vi "Partial Fraction Expansion.vi"(8 "option":u16(ring) items=["Cancel Co-factors", "Reserve Co-factors"], 9 "tolerance":dbl=1e-05, 10 "Denominator":cdb[](array[numeric]) format="%#.6g", 11 "Numerator":cdb[](array[numeric]) format="%#.6g") -> (0 "error":i32, 1 "Residues":cdb[][](array[numeric]) format="%#.6g", 2 "Poles":cdb[](array[numeric]) format="%#.6g", 3 "Polynomial":cdb[](array[numeric]) format="%#.6g", 5 "Multiplicity":i32[](array[numeric]))   [LabVIEW 2010, in "NI_AALPro.lvlib"]
doc: "Calculates the partial fraction expansion of a polynomial using the Heaviside cover-up method."
uses:
  NI_AALPro.lvlib
  Remove Zero Coefficients (CDB).vi
  Divide Polynomials (CDB).vi
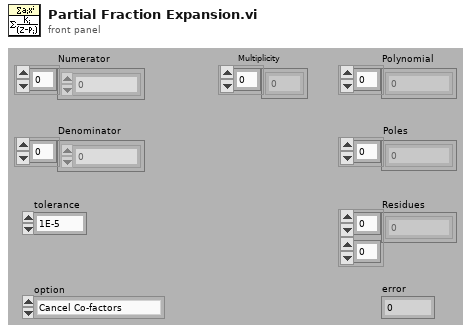
[diagram p1: front panel]
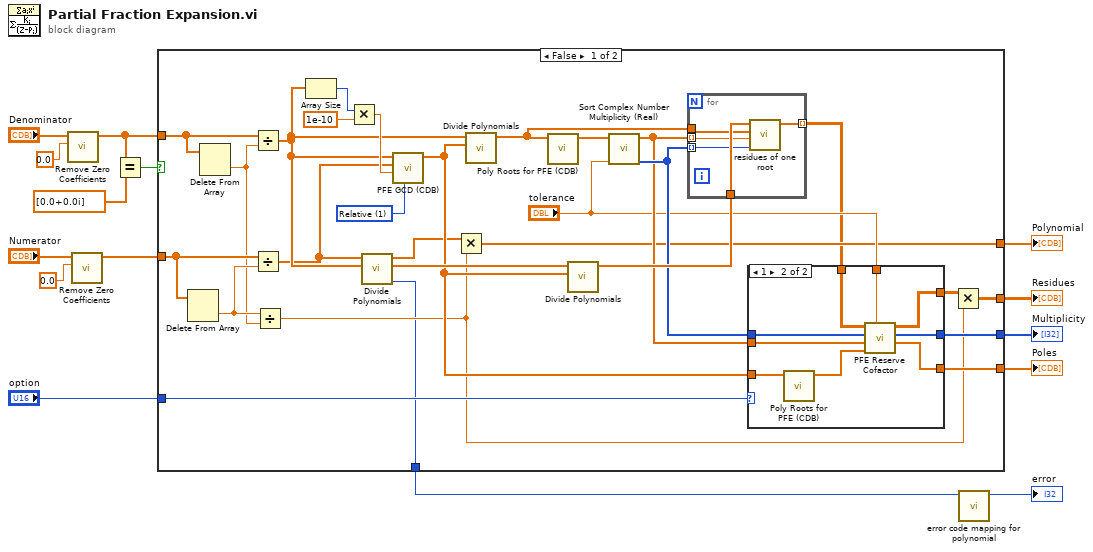
[diagram p0: block diagram]
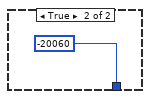
[diagram p3: hidden frame]
diagram:
  n1 = call-poly "Remove Zero Coefficients.vi"("threshold"=0.0, "P(x) In"="Denominator") -> ("P(x) Out"=w2:cdb[])  [unwired: 7 in, 2 out]
  n2 = call-poly "Remove Zero Coefficients.vi"("threshold"=0.0, "P(x) In"="Numerator") -> ("P(x) Out"=w8:cdb[])  [unwired: 7 in, 2 out]
  n3 = Equal?(x=w2, y=cdb[] [0.0+0.0i] ("P(x) Out")) -> (x = y?=w3:bool)
  n4 = case shown="False" w3 {
    tunnel: "option" -> [w39 _]
    tunnel: [w36 _] -> w10
    tunnel: [w35 _] -> w9
    tunnel: w2 -> [w29 _]
    tunnel: w8 -> [w27 _]
    tunnel: [w23 _] -> w7
    tunnel: [w17 _] -> w6
    tunnel: [w16 -20060] -> w4
    frame False {
      w30 = u16 1 items=["Absolute", "Relative"] ("tolerance type")
      n5 = Delete From Array(array=w27) -> (deleted portion=w25:cdb)  [unwired: 2 in, 1 out]
      n6 = Delete From Array(array=w29) -> (deleted portion=w24:cdb)  [unwired: 2 in, 1 out]
      n7 = Divide(x=w29, y=w24) -> (x/y=w28:cdb[])
      n8 = Divide(x=w27, y=w25) -> (x/y=w26:cdb[])
      n9 = Divide(x=w25, y=w24) -> (x/y=w18:cdb)
      n10 = Array Size(array=w28) -> (size(s)=w42:i32)
      n11 = Multiply(x=w42, y=1e-10 ("eps for GCD")) -> (x*y=w32:dbl)
      n12 = call-poly "Divide Polynomials.vi"("Q(x)"=w28, "P(x)"=w26) -> ("error"=w16:i32, "Remainder"=w41:cdb[], "P(x)/Q(x)"=w22:cdb[])  [unwired: 7 in]
      n13 = call "PFE GCD (CDB).vi"("tolerance type"=w30, "tolerance"=w32, "Q(x)"=w26, "P(x)"=w28) -> ("Greatest Common Divisor"=w31:cdb[])  [unwired: 6 in, 1 out]
      n14 = Multiply(x=w22, y=w18) -> (x*y=w23:cdb[])
      n15 = call-poly "Divide Polynomials.vi"("Q(x)"=w31, "P(x)"=w28) -> ("P(x)/Q(x)"=w21:cdb[])  [unwired: 7 in, 2 out]
      n16 = call "Poly Roots for PFE (CDB).vi"("P(x)"=w21) -> ("Roots"=w33:cdb[])  [unwired: 10 in]
      n17 = call-poly "Divide Polynomials.vi"("Q(x)"=w31, "P(x)"=w41) -> ("P(x)/Q(x)"=w40:cdb[])  [unwired: 7 in, 2 out]
      n18 = call "Sort Complex Number Multiplicity (Real).vi"("tolerance"="tolerance", "Complex numbers"=w33) -> ("Multiplicity"=w38:i32[], "Sorted unique complex numbers"=w37:cdb[])  [unwired: 8 in]
      n19 = for {
        tunnel: w38 -> [w57] mode=indexing
        tunnel: w37 -> [w58] mode=indexing
        tunnel: w40 -> [w60]
        tunnel: w21 -> [w59]
        tunnel: [w56] -> w20 mode=indexing
        n20 = call "residues of one root.vi"("multiplicity of root"=w57, "root"=w58, "Denominator"=w59, "Rest"=w60) -> ("Residues of root"=w56:cdb[])  [unwired: 7 in]
      }
      n21 = case shown="1" w39 {
        tunnel: w38 -> [w46 w54]
        tunnel: w37 -> [w45 w55]
        tunnel: [w45 w49] -> w36
        tunnel: [w46 w50] -> w35
        tunnel: w31 -> [_ w48]
        tunnel: w20 -> [w44 w53]
        tunnel: [w44 w51] -> w19
        tunnel: "tolerance" -> [_ w52]
        frame 0, Default {
        }
        frame 1 {
          n22 = call "Poly Roots for PFE (CDB).vi"("P(x)"=w48) -> ("Roots"=w47:cdb[])  [unwired: 10 in]
          n23 = call "PFE Reserve Cofactor.vi"("tolerance"=w52, "Co-factor Poles"=w47, "Poles In"=w55, "Multiplicity In"=w54, "Residues In"=w53) -> ("Poles Out"=w49:cdb[], "Multiplicity Out"=w50:i32[], "Residues Out"=w51:cdb[][])  [unwired: 4 in]
        }
      }
      n24 = Multiply(x=w19, y=w18) -> (x*y=w17:cdb[][])
    }
    frame True {
    }
  }
  "Poles" <- w10
  "Multiplicity" <- w9
  "Residues" <- w6
  "Polynomial" <- w7
  n25 = call "error code mapping for polynomial.vi"("error in"=w4) -> ("error out"=→"error":i32)  [unwired: 10 in]
